vi "Generate Report.vi"(8 "error in (no error)":errorcluster, 10 "Resource In":variant, 11 "HIJ IMAQdx Display in":refnum<class "HIJ IMAQdx Display.lvclass">) -> (0 "error out":errorcluster, 2 "Resource Out":variant, 3 "HIJ IMAQdx Display out":refnum<class "HIJ IMAQdx Display.lvclass">)   [LabVIEW 2014, in "HIJ IMAQdx Display.lvlib" / "HIJ IMAQdx Display.lvclass"]
uses:
  HIJ IMAQdx Display.lvclass
  HIJ Vision Display/HIJ Vision Display/HIJ Vision Display.lvclass/HIJ Vision Display.ctl
  <vilib>/ActorFramework/Message Enqueuer/Message Priority.ctl
  HIJ Vision Display/HIJ Vision Display/Read Image Source.vi
  HIJ Vision Display/HIJ Vision Display/HIJ Vision Display.lvclass
  <vilib>/ActorFramework/Message Enqueuer/Message Enqueuer.lvclass
  Camera Actor/Camera Actor Messages/Write Settings to Ini File/Write Settings to Ini File.lvclass
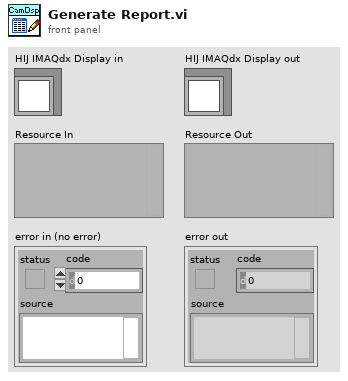
[diagram p1: front panel]
types:
  T1 = typedef "Actor Framework.lvlib/Message Enqueuer.lvclass/Message Priority.ctl" = enum16{"Low", "Normal", "High"}
  T2 = typedef "NI_LVConfig.lvlib/Config Data RefNum.ctl" = refnum<k1>
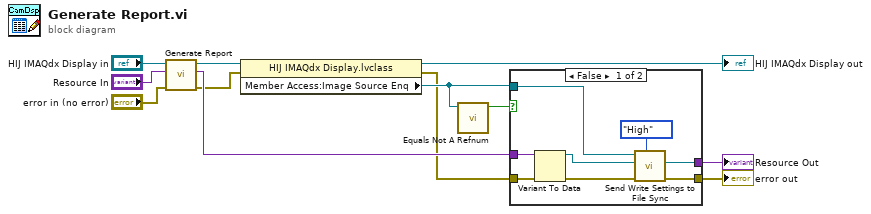
[diagram p0: block diagram]
diagram:
  n1 = call-parent "Generate Report.vi"("error in (no error)"="error in (no error)", "Resource In"="Resource In", "HIJ Vision Display in"="HIJ IMAQdx Display in") -> ("error out"=w4:errorcluster, "Resource Out"=w7:variant, "HIJ Vision Display out"=w12:refnum<class "HIJ IMAQdx Display.lvclass">)  [unwired: 6 in]
  n2 = property class="HIJ IMAQdx Display.lvclass"(reference=w12, error in=w4) -> (reference out=→"HIJ IMAQdx Display out":refnum<class "HIJ IMAQdx Display.lvclass">, error out=w2:errorcluster, "Member Access:Image Source Enq"=w3:refnum<class "Message Enqueuer.lvclass">)
  n3 = call <vilib>:"Equals Not A Refnum.vi"("Message Enqueuer"=w3) -> ("Not a refnum?"=w1:bool)  [unwired: 10 in]
  n4 = case shown="False" w1 {
    tunnel: w7 -> [w19 w22]
    tunnel: [w16 w21] -> w6
    tunnel: [w15 w22] -> w5
    tunnel: w3 -> [w14 _]
    tunnel: w2 -> [w13 w21]
    frame False {
      n5 = Variant To Data(error in=w13, Variant=w19) -> (data=w18:T2, error out=w17:errorcluster)  [unwired: 1 in]
      n6 = call "Send Write Settings to File Sync.vi"("Message Priority (Normal)"=Message_Priority."High", "error in (no error)"=w17, "file refnum"=w18, "Message Enqueuer in"=w14) -> ("error out"=w16:errorcluster, "file ref"=w15:T2)  [unwired: 4 in, 2 out]
    }
    frame True {
    }
  }
  "error out" <- w6
  "Resource Out" <- w5
